vi "New DB.vi"(8 "error in (no error)":errorcluster, 11 "SQLite Database in":refnum<class "SQLite Database.lvclass">) -> (0 "error out":errorcluster, 3 "SQLite Database out":refnum<class "SQLite Database.lvclass">)   [LabVIEW 2019, in "TSC Event Logger.lvlib" / "SQLite Database.lvclass"]
doc: "Create a SQLite database sink.\n\n<b>Code Developed By:</b>\nTechnology Service Corporation\nBloomington, IN 47403\nwww.tsc.com/atcs\n\nDeveloper:\nDaniel Coons"
uses:
  SQLite Database.lvclass
  SQLite Database.lvclass/SQLite Database.ctl
  <vilib>/drjdpowell/SQLite Library/SQL Connection/Open (path).vi
  <vilib>/drjdpowell/SQLite Library/SQL Connection/Open (string).vi
  <vilib>/AdvancedString/Path To Command Line String.vi
  <vilib>/drjdpowell/SQLite Library/SQL Connection/Execute SQL (No results).vi
  <vilib>/drjdpowell/SQLite Library/SQL Connection/Connection.lvclass
  <vilib>/drjdpowell/SQLite Library/SQLite.lvlib
  Log Sinks.lvclass
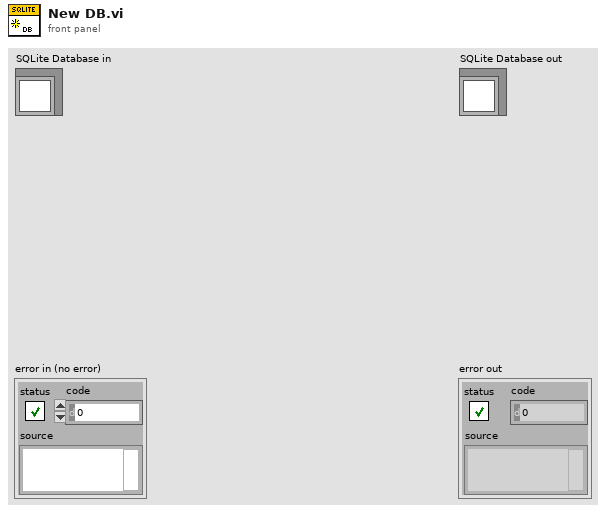
[diagram p1: front panel]
types:
  T1 = enum16{"New or existing", "Existing", "Read only"}
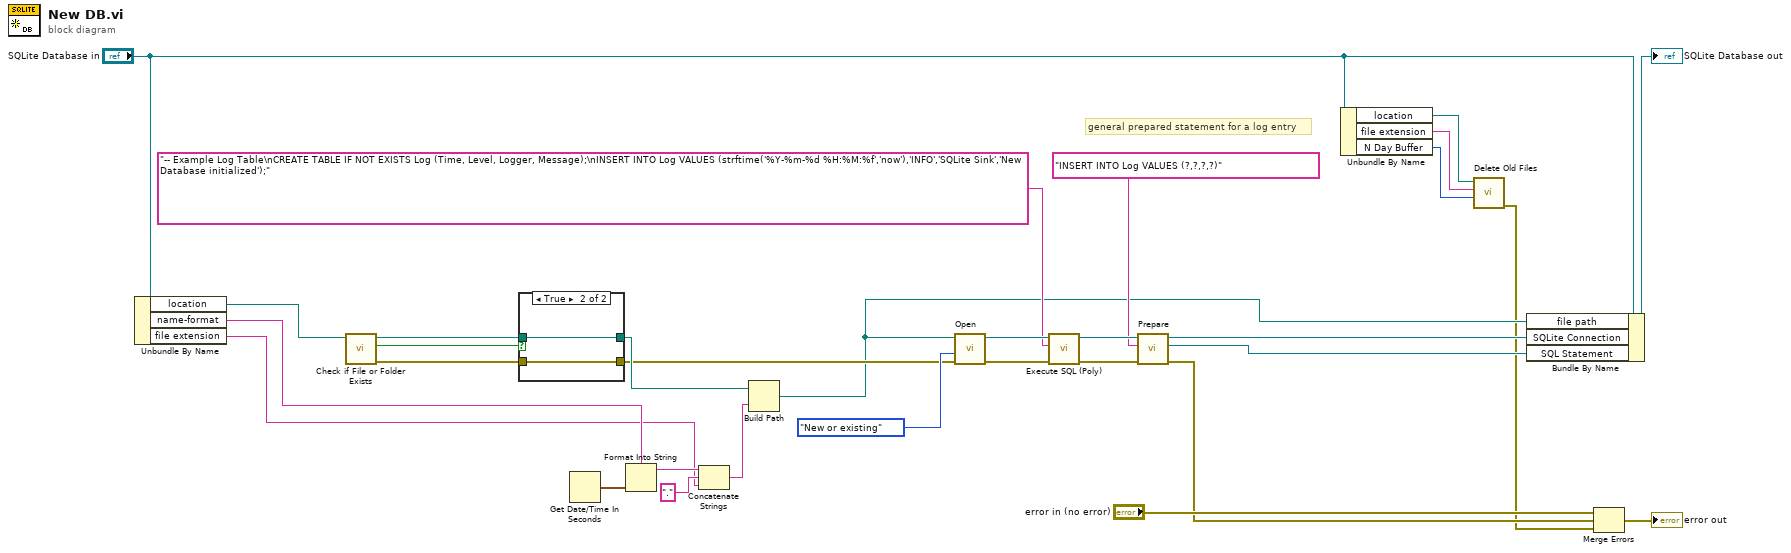
[diagram p0: block diagram]
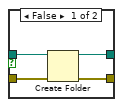
[diagram p2: hidden frame]
diagram:
  # "general prepared statement for a log entry"
  n1 = Unbundle By Name("SQLite Database in") -> ("location"=w22:path, "name-format"=w21:string, "file extension"=w20:string)
  n2 = call <vilib>:"Check if File or Folder Exists.vi"("path"=w22) -> ("error out"=w24:errorcluster, "file or folder exists?"=w25:bool, "dup path"=w26:path)  [unwired: 8 in]
  n3 = case shown="True" w25 {
    tunnel: w26 -> [w35 w37]
    tunnel: [w34 w37] -> w23
    tunnel: w24 -> [w33 w36]
    tunnel: [w32 w36] -> w16
    frame False {
      n4 = Create Folder(path (use dialog)=w35, error in=w33) -> (created path=w34:path, error out=w32:errorcluster)  [unwired: 1 in, 1 out]
    }
    frame True {
    }
  }
  n5 = Get Date/Time In Seconds() -> (seconds since 1Jan1904=w29:timestamp)
  n6 = Format Into String(format string=w21, w29) -> (resulting string=w30:string)  [unwired: 2 in, 1 out]
  n7 = Concatenate Strings(w30, "." ("string"), w20) -> (w28:string)
  n8 = Build Path(base path=w23, name or relative path=w28) -> (appended path=w6:path)
  n9 = call-poly <vilib>:"Open.vi"("error in (no error)"=w16, "File Option"=T1."New or existing", "db file"=w6) -> ("error out"=w15:errorcluster, "SQLite Connection"=w14:refnum<class "Connection.lvclass">)  [unwired: 7 in]
  n10 = call-poly <vilib>:"Execute SQL (Poly).vi"("error in (no error)"=w15, "SQL"="-- Example Log Table\nCREATE TABLE IF NOT EXISTS Log (Time, Level, Logger, Message);\nINSERT INTO Log VALUES (strftime('%Y-%m-%d %H:%M:%f','now'),'INFO','SQLite Sink','New Database initialized');", "SQLite Connection in"=w14) -> ("error out"=w13:errorcluster, "SQLite Connection"=w11:refnum<class "Connection.lvclass">)  [unwired: 7 in]
  n11 = call <vilib>:"Prepare.vi"("error in (no error)"=w13, "SQL"="INSERT INTO Log VALUES (?,?,?,?)", "SQLite Connection in"=w11) -> ("error out"=w12:errorcluster, "SQL Statement"=w8:refnum<class "SQL Statement.lvclass">, "SQLite Connection"=w10:refnum<class "Connection.lvclass">)  [unwired: 4 in, 2 out]
  n12 = Unbundle By Name("SQLite Database in") -> ("location"=w3:path, "file extension"=w4:string, "N Day Buffer"=w5:u32)
  n13 = call "Delete Old Files.vi"("N Day Buffer"=w5, "file extension"=w4, "location"=w3) -> ("error out"=w1:errorcluster)  [unwired: 8 in]
  n14 = Bundle By Name(cluster="SQLite Database in", "file path"=w6, "SQLite Connection"=w10, "SQL Statement"=w8) -> (→"SQLite Database out":refnum<class "SQLite Database.lvclass">)
  n15 = Merge Errors("error in (no error)", w12, w1) -> (→"error out":errorcluster)
